vi "runTestScenario.vi"(8 "error in (no error)":errorcluster, 11 "Constant Analog Output Voltage Test  in":refnum<class "Constant Analog Output Voltage Test.lvclass">) -> (0 "error out":errorcluster, 1 "Result":T1, 2 "TestExecution":T2, 3 "Constant Analog Output Voltage Test  out":refnum<class "Constant Analog Output Voltage Test.lvclass">)   [LabVIEW 2015, in "Constant Analog Output Voltage Test.lvclass"]
uses:
  Constant Analog Output Voltage Test.lvclass
  Typedefs/TestExecution.ctl
  Typedefs/PassFailTest.ctl
  Typedefs/WriteDataFileInput.ctl
  Typedefs/TestScenarioTypes.ctl
  Typedefs/WriteLogMessageInput.ctl
  Constant Analog Output Voltage Test.lvclass/Constant Analog Output Voltage Test.ctl
  Model/TestLog/ITestLog/ITestLog.lvclass
  Typedefs/ILCBTTypedefs.lvlib
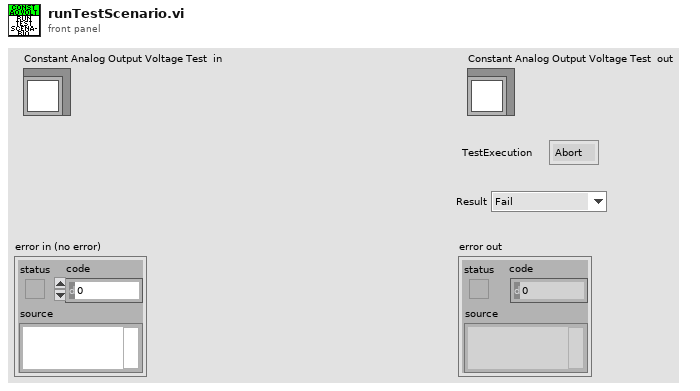
[diagram p1: front panel]
types:
  T1 = typedef "ILCBTTypedefs.lvlib/PassFailTest.ctl" = enum16{"Fail", "Pass", "NA"}
  T2 = typedef "ILCBTTypedefs.lvlib/TestExecution.ctl" = enum16{"Abort", "Continue"}
  T3 = typedef "ILCBTTypedefs.lvlib/WriteLogMessageInput.ctl" = cluster{"Test Scenario":T4, "Description":string, "Actual Value":string, "Data File":string, "Result":T1}
  T4 = typedef "ILCBTTypedefs.lvlib/TestScenarioTypes.ctl" = enum16{"+3.3VA Supply Test", "+3.3VD Supply Test", "+5VA Supply Test", "+5VD Supply Test", "Unique ID Test", "TEDS Status Test", "LIMSW1_TTL Low Test", "LIMSW1_TTL High Test", "LIMSW2_TTL Low Test", "LIMSW2_TTL High Test", "Tachometer Low Test", "Tachometer High Test", "SSR_TTL Low Test", "SSR_TTL High Test", "SM_GPI Low Test", "SM_GPI High Test", "CW Motion Without Limit Test", "CW Motion With Limit Test", "CW Motion With Both Limits Test", "CW Motion on CCW Limit Test", "CCW Motion Without Limit Test", "CCW Motion With Limit Test", "CCW Motion With Both Limits Test", "CCW Motion on CW Limit Test", "RS232-TXD Low Test", "RS232-TXD High Test", "RS232-RTS Low Test", "RS232-RTS High Test", "RS232-RXD Low Test", "RS232-RXD High Test", "RS232-CTS Low Test", "RS232-CTS High Test", "Out_SS Low Test", "Out_SS High Test", "Out_SDI Low Test", "Out_SDI High Test", "Out_SCLK Low Test", "Out_SCLK High Test", "Reset Low Test", "Reset High Test", "1 Channel ADC Test", "3 Channel ADC Test", "5 Channel ADC Test", "Vref Test", "ROT Test", "DAC1 Test", "DAC2 Test", "DAC3 Test", "DAC4 Test", "BIAS Test", "EXC1 Test", "EXC2 Test", "EXC3 Test", "EXC4 Test"}
  T5 = typedef "ILCBTTypedefs.lvlib/WriteDataFileInput.ctl" = cluster{"Test Scenario":T4, "File Name":string, "Output":string[]}
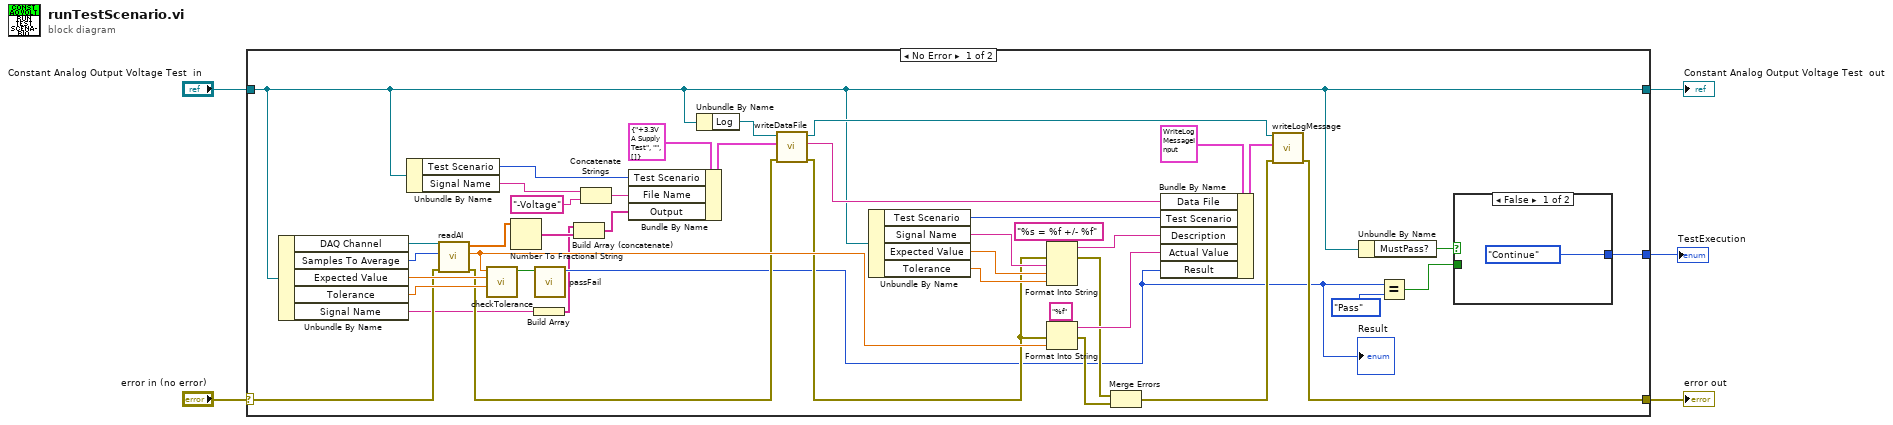
[diagram p0: block diagram]
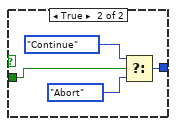
[diagram p2: hidden frame]
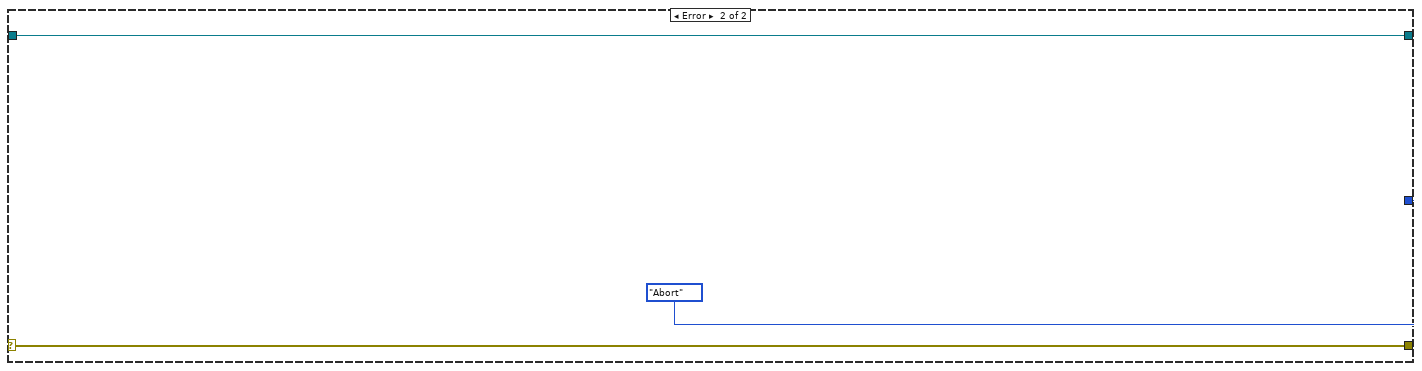
[diagram p3: hidden frame]
diagram:
  n1 = case shown="No Error" "error in (no error)" {
    selector: "error in (no error)" -> [w24 w56]
    tunnel: [w19 w56] -> w4
    tunnel: [w15 TestExecution."Abort" ("TestExecution")] -> w3
    tunnel: "Constant Analog Output Voltage Test  in" -> [w17 w54]
    tunnel: [w17 w54] -> w1
    frame No Error {
      n2 = Unbundle By Name(w17) -> ("DAQ Channel"=w48:refnum<k21>, "Samples To Average"=w41:i32, "Expected Value"=w40:dbl, "Tolerance"=w39:dbl, "Signal Name"=w7:string)
      n3 = Unbundle By Name(w17) -> ("Test Scenario"=w44:T4, "Signal Name"=w43:string)
      n4 = call "readAI.vi"("error in (no error)"=w24, "Samples To Read"=w41, "DAQ Channel To Read"=w48) -> ("error out"=w23:errorcluster, "Average"=w27:dbl, "Samples"=w12:dbl[])  [unwired: 6 in]
      n5 = call "checkTolerance.vi"("Tolerance"=w39, "Expected Value"=w40, "Average"=w27) -> ("Boolean"=w36:bool)  [unwired: 8 in]
      n6 = Number To Fractional String(number=w12) -> (F-format string=w9:string[])  [unwired: 3 in]
      n7 = Build Array(w7) -> (w6:string[])
      n8 = call "passFail.vi"("Boolean"=w36) -> ("Result"=w11:T1)  [unwired: 10 in]
      "Result" <- w11
      n9 = Build Array (concatenate)(w6, w9) -> (w8:string[])
      n10 = Concatenate Strings(w43, "-Voltage" ("string")) -> (w42:string)
      n11 = Bundle By Name(cluster=T5 {"Test Scenario"=enum."+3.3VA Supply Test", "File Name"="", "Output"=[]} ("WriteDataFileInput"), "Test Scenario"=w44, "File Name"=w42, "Output"=w8) -> (w45:T5)
      n12 = Unbundle By Name(w17) -> ("Log"=w47:refnum<class "ITestLog.lvclass">)
      n13 = call-dynamic "writeDataFile.vi"("error in (no error)"=w23, "WriteDataFileInput"=w45, "ITestLog in"=w47) -> ("error out"=w18:errorcluster, "Relative Path"=w35:string, "ITestLog out"=w25:refnum<class "ITestLog.lvclass">)  [unwired: 6 in]
      n14 = Unbundle By Name(w17) -> ("Test Scenario"=w34:T4, "Signal Name"=w32:string, "Expected Value"=w31:dbl, "Tolerance"=w30:dbl)
      n15 = Format Into String(format string="%s = %f +/- %f", error in=w18, w32, w31, w30) -> (resulting string=w29:string, error out=w22:errorcluster)  [unwired: 1 in]
      n16 = Format Into String(format string="%f", error in=w18, w27) -> (resulting string=w26:string, error out=w21:errorcluster)  [unwired: 1 in]
      n17 = Merge Errors(w22, w21) -> (w20:errorcluster)
      n18 = Bundle By Name(cluster=T3 {"Test Scenario"=enum."+3.3VA Supply Test", "Description"="", "Actual Value"="", "Data File"="", "Result"=enum."Fail"} ("WriteLogMessageInput"), "Data File"=w35, "Test Scenario"=w34, "Description"=w29, "Actual Value"=w26, "Result"=w11) -> (w37:T3)
      n19 = call-dynamic "writeLogMessage.vi"("error in (no error)"=w20, "WriteLogMessageInput"=w37, "ITestLog in"=w25) -> ("error out"=w19:errorcluster)  [unwired: 7 in, 1 out]
      n20 = Unbundle By Name(w17) -> ("MustPass?"=w16:bool)
      n21 = Equal?(x=w11, y=PassFailTest."Pass") -> (x = y?=w13:bool)
      n22 = case shown="False" w16 {
        tunnel: [TestExecution."Continue" ("TestExecution") w53] -> w15
        tunnel: w13 -> [_ w50]
        frame False {
        }
        frame True {
          n23 = Select(t=TestExecution."Continue" ("TestExecution"), s=w50, f=TestExecution."Abort" ("TestExecution")) -> (s? t:f=w53:T2)
        }
      }
    }
    frame Error {
    }
  }
  "Constant Analog Output Voltage Test  out" <- w1
  "error out" <- w4
  "TestExecution" <- w3
